vi "Set_FAMM_class.vi"(8 "error in (no error)":errorcluster, 10 "FAMM.lvclass":refnum<class "FAMM.lvclass">, 11 "Vsolver in":refnum<class "Vsolver.lvclass">) -> (0 "error out":errorcluster, 3 "Vsolver out":refnum<class "Vsolver.lvclass">)   [LabVIEW 2020, in "Vsolver.lvclass"]
doc: "Set FAMM class\n\nThis method should only be used by Gserver"
uses:
  Vsolver.lvclass
  FAMM/FAMM.lvclass
  Vsolver.lvclass/Vsolver.ctl
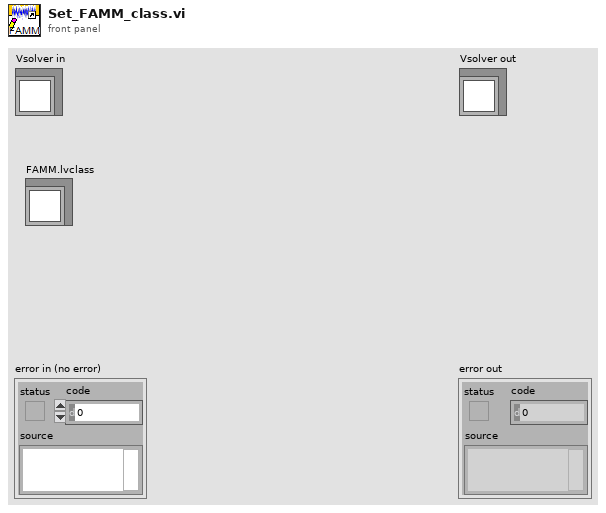
[diagram p1: front panel]
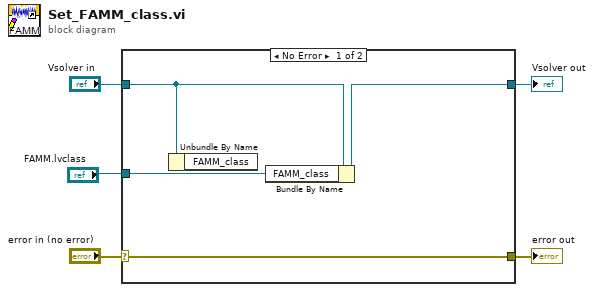
[diagram p0: block diagram]
diagram:
  n1 = case shown="No Error" "error in (no error)" {
    selector: "error in (no error)" -> [w9 w10]
    tunnel: [w9 w10] -> w4
    tunnel: [w8 w11] -> w2
    tunnel: "Vsolver in" -> [w6 w11]
    tunnel: "FAMM.lvclass" -> [w7 _]
    frame No Error {
      n2 = Unbundle By Name(w6) -> ()  [unwired: 1 out]
      n3 = Bundle By Name(cluster=w6, "FAMM_class"=w7) -> (w8:refnum<class "Vsolver.lvclass">)
    }
    frame Error {
    }
  }
  "error out" <- w4
  "Vsolver out" <- w2
